vi "labSSH_FGGA_Files_Transfer.vi"(0 "Flight_num":string, 1 "Get current?":bool, 5 "Date":string, 7 "Flight Folder Path":path) -> (15 "error IO":errorcluster)   [LabVIEW 2014]
uses:
  <vilib>/Labwerx/labSSH/labSSH.lvlib
panel:
  out "Array of Directory Entries":T1(array[cluster]) {"File Info"."Permissions" format="%o"}
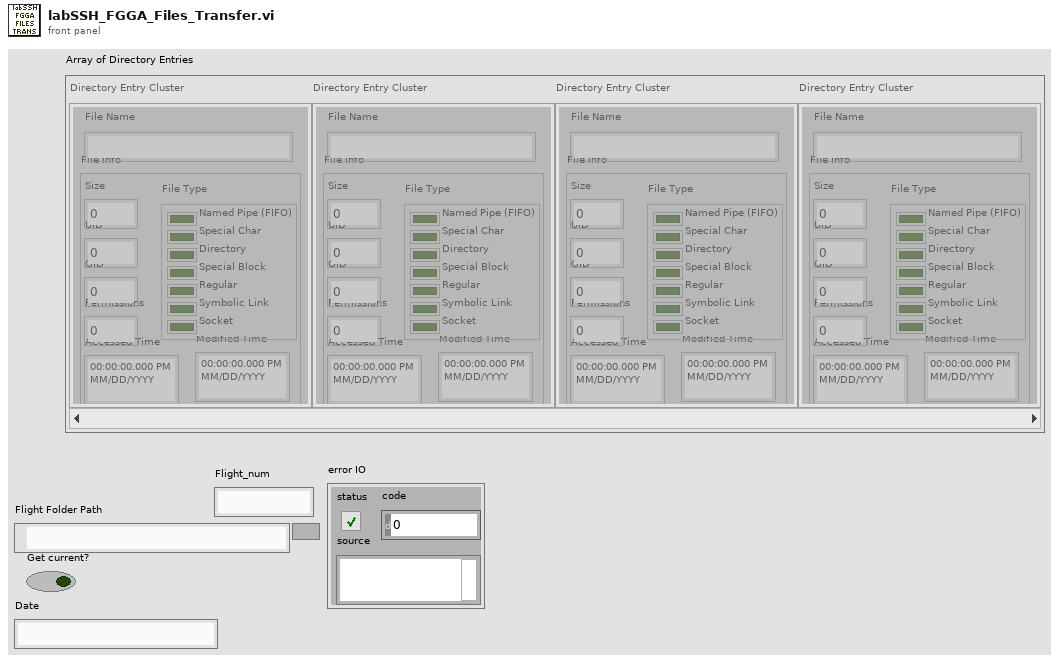
[diagram p1: front panel]
types:
  T1 = cluster{"File Info":cluster{"Size":u32, "UID":u32, "GID":u32, "Permissions":u32, "Accessed Time":timestamp, "Modified Time":timestamp, "File Type":cluster{"Socket":bool, "Directory":bool, "Special Char":bool, "Special Block":bool, "Symbolic Link":bool, "Regular":bool, "Named Pipe (FIFO)":bool}}, "File Name":string}[]
  T2 = enum32{"invalid app kind", "Development System", "Run Time System", "Student Edition", "Embedded LabVIEW", "Evaluation", "Custom"}
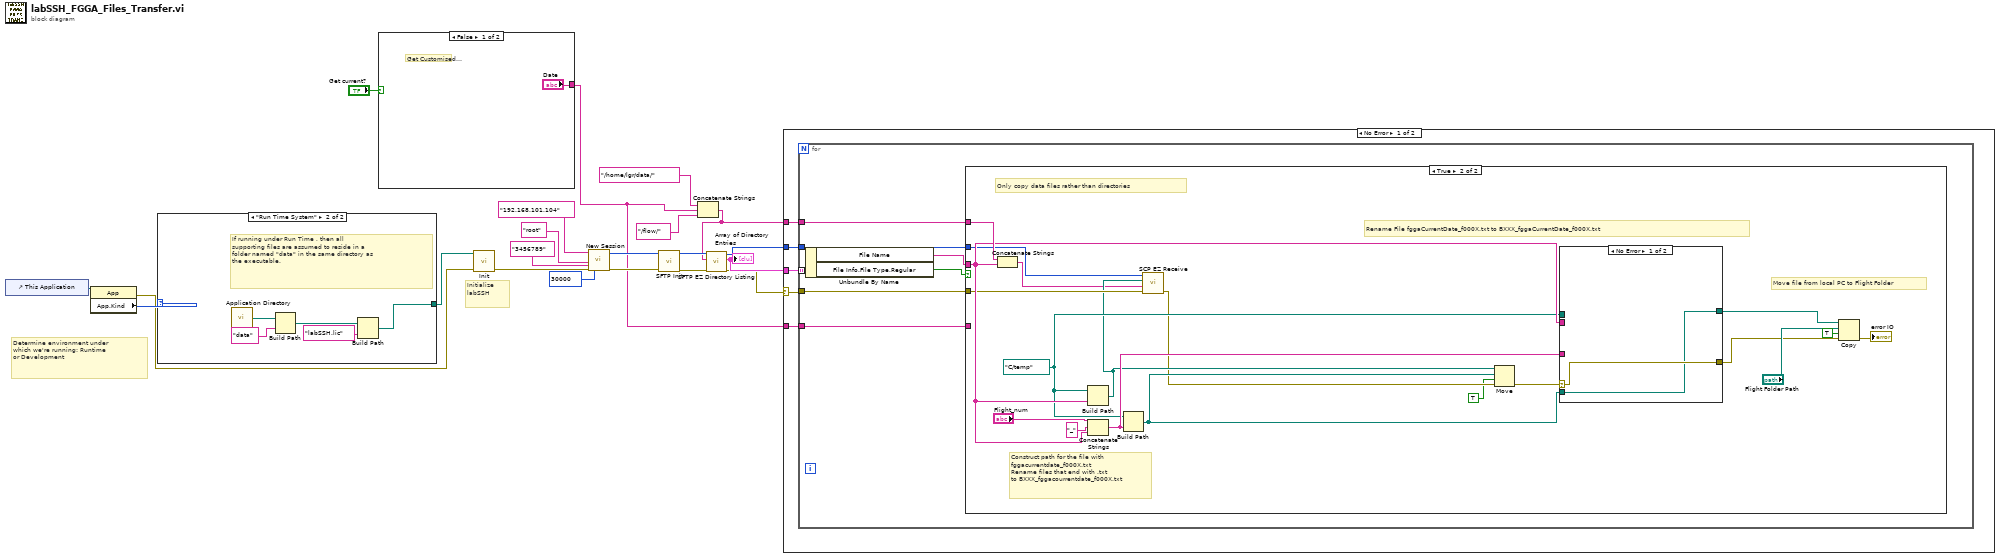
[diagram p0: block diagram]
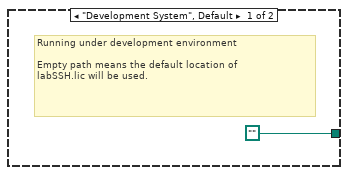
[diagram p2: hidden frame]
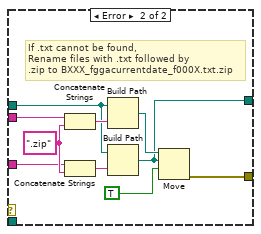
[diagram p4: hidden frame]
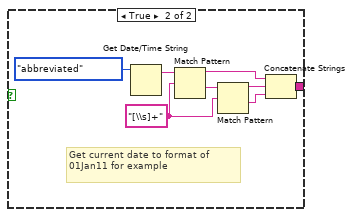
[diagram p6: hidden frame]
diagram:
  # "Initialize \nlabSSH"
  # "Determine environment under\nwhich we're running: Runtime\nor Development"
  n1 = control-ref of="This Application"() -> (w5:refnum<vi>)
  n2 = property class="App"(reference=w5) -> (error out=w2:errorcluster, "App.Kind"=w4:T2)  [unwired: 1 in, 1 out]
  n3 = case shown="\"Run Time System\"" w4 {
    tunnel: [path "" w24] -> w3
    frame "Development System", Default {
      # "Running under development environment\n\nEmpty path means the default location of\nlabSSH.lic will be used."
    }
    frame "Run Time System" {
      # "If running under Run Time , then all\nsupporting files are assumed to reside in a \nfolder named \"data\" in the same directory as\nthe executable."
      n4 = call <vilib>:"Application Directory.vi"() -> ("Application Directory"=w23:path)
      n5 = Build Path(base path=w23, name or relative path="data") -> (appended path=w25:path)
      n6 = Build Path(base path=w25, name or relative path="labSSH.lic") -> (appended path=w24:path)
    }
  }
  n7 = case shown="False" "Get current?" {
    tunnel: ["Date" w29] -> w6
    frame False {
      # "Get Customised Date"
    }
    frame True {
      w34 = "[\\s]+" ("regular expression")
      # "Get current date to format of\n01Jan11 for example"
      n8 = Get Date/Time String(date format (0)=enum16{"short", "long", "abbreviated"}."abbreviated") -> (date string=w35:string)  [unwired: 2 in, 1 out]
      n9 = Match Pattern(string=w35, regular expression=w34) -> (before substring=w32:string, after substring=w33:string)  [unwired: 1 in, 2 out]
      n10 = Match Pattern(string=w33, regular expression=w34) -> (before substring=w31:string, after substring=w30:string)  [unwired: 1 in, 2 out]
      n11 = Concatenate Strings(w32, w31, w30) -> (w29:string)
    }
  }
  n12 = call <vilib>:"Init.vi"("error in (no error)"=w2, "License File Path Override"=w3) -> ("error out"=w21:errorcluster)  [unwired: 9 in]
  n13 = call <vilib>:"New Session.vi"("IP Addr or Hostname"="192.168.101.104", "Username"="root", "Password"="3456789", "error in (no error)"=w21, "Timeout msec (10000)"=30000) -> ("New LabSSH Session"=w16:u64, "error out"=w17:errorcluster)  [unwired: 13 in]
  n14 = call <vilib>:"SFTP Init.vi"("error in (no error)"=w17, "LabSSH Session"=w16) -> ("error out"=w14:errorcluster, "LabSSH Session Out"=w15:u64)  [unwired: 8 in]
  n15 = Concatenate Strings("/home/lgr/data/" ("string"), w6, "/flow/" ("string")) -> (w9:string)
  n16 = call <vilib>:"SFTP EZ Directory Listing.vi"("error in (no error)"=w14, "Remote Directory Path"=w9, "LabSSH Session"=w15) -> ("error out"=w7:errorcluster, "Array of Directory Entries"=w11:T1, "LabSSH Session Out"=w10:u64)  [unwired: 5 in, 1 out]
  "Array of Directory Entries" <- w11
  n17 = case shown="No Error" w7 {
    selector: w7 -> [w38 _]
    tunnel: w11 -> [w41 _]
    tunnel: w10 -> [w40 _]
    tunnel: w9 -> [w39 _]
    tunnel: w6 -> [w37 _]
    frame No Error {
      n18 = for {
        tunnel: w41 -> [w48] mode=indexing
        tunnel: w40 -> [w47]
        tunnel: w38 -> [w46]
        tunnel: w39 -> [w45]
        tunnel: w37 -> [w43]
        n19 = Unbundle By Name(w48) -> ("File Name"=w44:string, "File Info.File Type.Regular"=w42:bool)
        n20 = case shown="True" w42 {
          tunnel: w47 -> [_ w59]
          tunnel: w46 -> [_ w60]
          tunnel: w45 -> [_ w67]
          tunnel: w44 -> [_ w63]
          tunnel: w43 -> [_ _]
          frame False {
          }
          frame True {
            w62 = path "C:/temp" ("working directory")
            # "Move file from local PC to Flight Folder"
            # "Rename File fggaCurrentDate_f000X.txt to BXXX_fggaCurrentDate_f000X.txt"
            # "Construct path for the file with\nfggacurrentdate_f000X.txt\nRename files that end with .txt\nto BXXX_fggacourrentdate_f000X.txt"
            # "Only copy data files rather than directories"
            n21 = Concatenate Strings(w67, w63) -> (w57:string)
            n22 = Build Path(base path=w62, name or relative path=w63) -> (appended path=w58:path)
            n23 = Concatenate Strings("Flight_num", "_" ("string"), w63) -> (w65:string)
            n24 = Build Path(base path=w62, name or relative path=w65) -> (appended path=w61:path)
            n25 = call <vilib>:"SCP EZ Receive.vi"("error in (no error)"=w60, "Remote Path"=w57, "Local Path"=w58, "LabSSH Session"=w59) -> ("error out"=w56:errorcluster)  [unwired: 3 in, 3 out]
            n26 = Move(source path=w58, error in=w56, 9:TRUE ("overwrite (F)"), 10:w61) -> (error out=w51:errorcluster)  [unwired: 1 in, 2 out]
            n27 = case shown="No Error" w51 {
              selector: w51 -> [w69 _]
              tunnel: w63 -> [_ w79]
              tunnel: w65 -> [_ w75]
              tunnel: [w69 w73] -> w54
              tunnel: [w68 w72] -> w53
              tunnel: w61 -> [w68 _]
              tunnel: w62 -> [_ w70]
              frame No Error {
              }
              frame Error {
                w76 = ".zip" ("string")
                # "If .txt cannot be found,\nRename files with .txt followed by\n.zip to BXXX_fggacurrentdate_f000X.txt.zip"
                n28 = Concatenate Strings(w79, w76) -> (w78:string)
                n29 = Concatenate Strings(w75, w76) -> (w74:string)
                n30 = Build Path(base path=w70, name or relative path=w78) -> (appended path=w77:path)
                n31 = Build Path(base path=w70, name or relative path=w74) -> (appended path=w72:path)
                n32 = Move(source path=w77, 9:TRUE ("overwrite (F)"), 10:w72) -> (error out=w73:errorcluster)  [unwired: 2 in, 2 out]
              }
            }
            n33 = Copy(8:w54, 9:TRUE ("overwrite (F)"), 10:"Flight Folder Path", 11:w53) -> (0:→"error IO":errorcluster)  [unwired: 1 in, 2 out]
          }
        }
      }
    }
    frame Error {
    }
  }
